vi "球体体积.vi"(11 "Radious":dbl) -> (3 "Area":dbl=nan)   [LabVIEW 2011]
doc: "功能：\n计算球体体积。\n\n公式：\ns=4/3*Pi*r^3\n\ncsxcs_366创建"
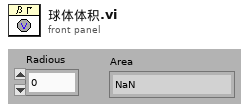
[diagram p1: front panel]
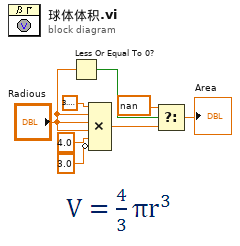
[diagram p0: block diagram]
diagram:
  n1 = Less Or Equal To 0?(x="Radious") -> (x <= 0?=w8:bool)
  n2 = Compound Arithmetic op=MULTIPLY(3.141592653589793, "Radious", "Radious", "Radious", 4.0 ("值"), invert 3.0 ("值")) -> (w5:dbl)
  n3 = Select(t=nan, s=w8, f=w5) -> (s? t:f=→"Area":dbl)
